vi "UpdateExpFile.vi"(3 "ExpFilePath":path) -> (1 "error out":errorcluster)   [LabVIEW 2013]
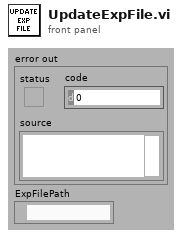
[diagram p1: front panel]
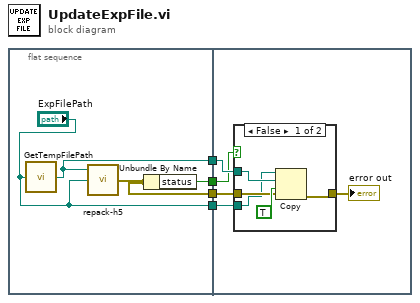
[diagram p0: block diagram]
diagram:
  n1 = flat-sequence {
    tunnel: [w6] -> w4
    tunnel: ["ExpFilePath"] -> w3
    tunnel: [w7] -> w2
    tunnel: [w8] -> w1
    tunnel: w4 -> [w11]
    tunnel: w3 -> [w13]
    tunnel: w2 -> [w12]
    tunnel: w1 -> [w10]
    frame #0 {
      n2 = call "GetTempFilePath.vi"("ExpFilePath"="ExpFilePath") -> ("Temp file path"=w6:path)
      n3 = call "repack-h5.vi"("dest"="ExpFilePath", "source"=w6) -> ("error out"=w7:errorcluster)  [unwired: 1 in]
      n4 = Unbundle By Name(w7) -> ("status"=w8:bool)
    }
    frame #1 {
      n5 = case shown="False" w10 {
        tunnel: w13 -> [w14 _]
        tunnel: w12 -> [w16 w19]
        tunnel: [w18 w19] -> w9
        tunnel: w11 -> [w15 _]
        frame False {
          n6 = Copy(8:w16, 9:TRUE, 10:w15, 11:w14) -> (0:w18:errorcluster)  [unwired: 1 in, 2 out]
        }
        frame True {
        }
      }
      "error out" <- w9
    }
  }
